vi "Digital input.vi"(8 "error in":errorcluster, 11 "DAQmx InPut Setting":T1) -> (0 "error out":errorcluster, 1 "Exit":bool)   [LabVIEW 2015]
uses:
  <vilib>/DAQmx/read.llb/DAQmx Read (Digital 1D Bool 1Chan 1Samp).vi
  <vilib>/DAQmx/create/channels.llb/DAQmx Create Channel (DI-Digital Input).vi
  Galobal variable_TI.vi
  <vilib>/DAQmx/miscellaneous.llb/DAQmx Fill In Error Info.vi
panel:
  in  "Count":i32
  out "Array":bool[](array[boolean])
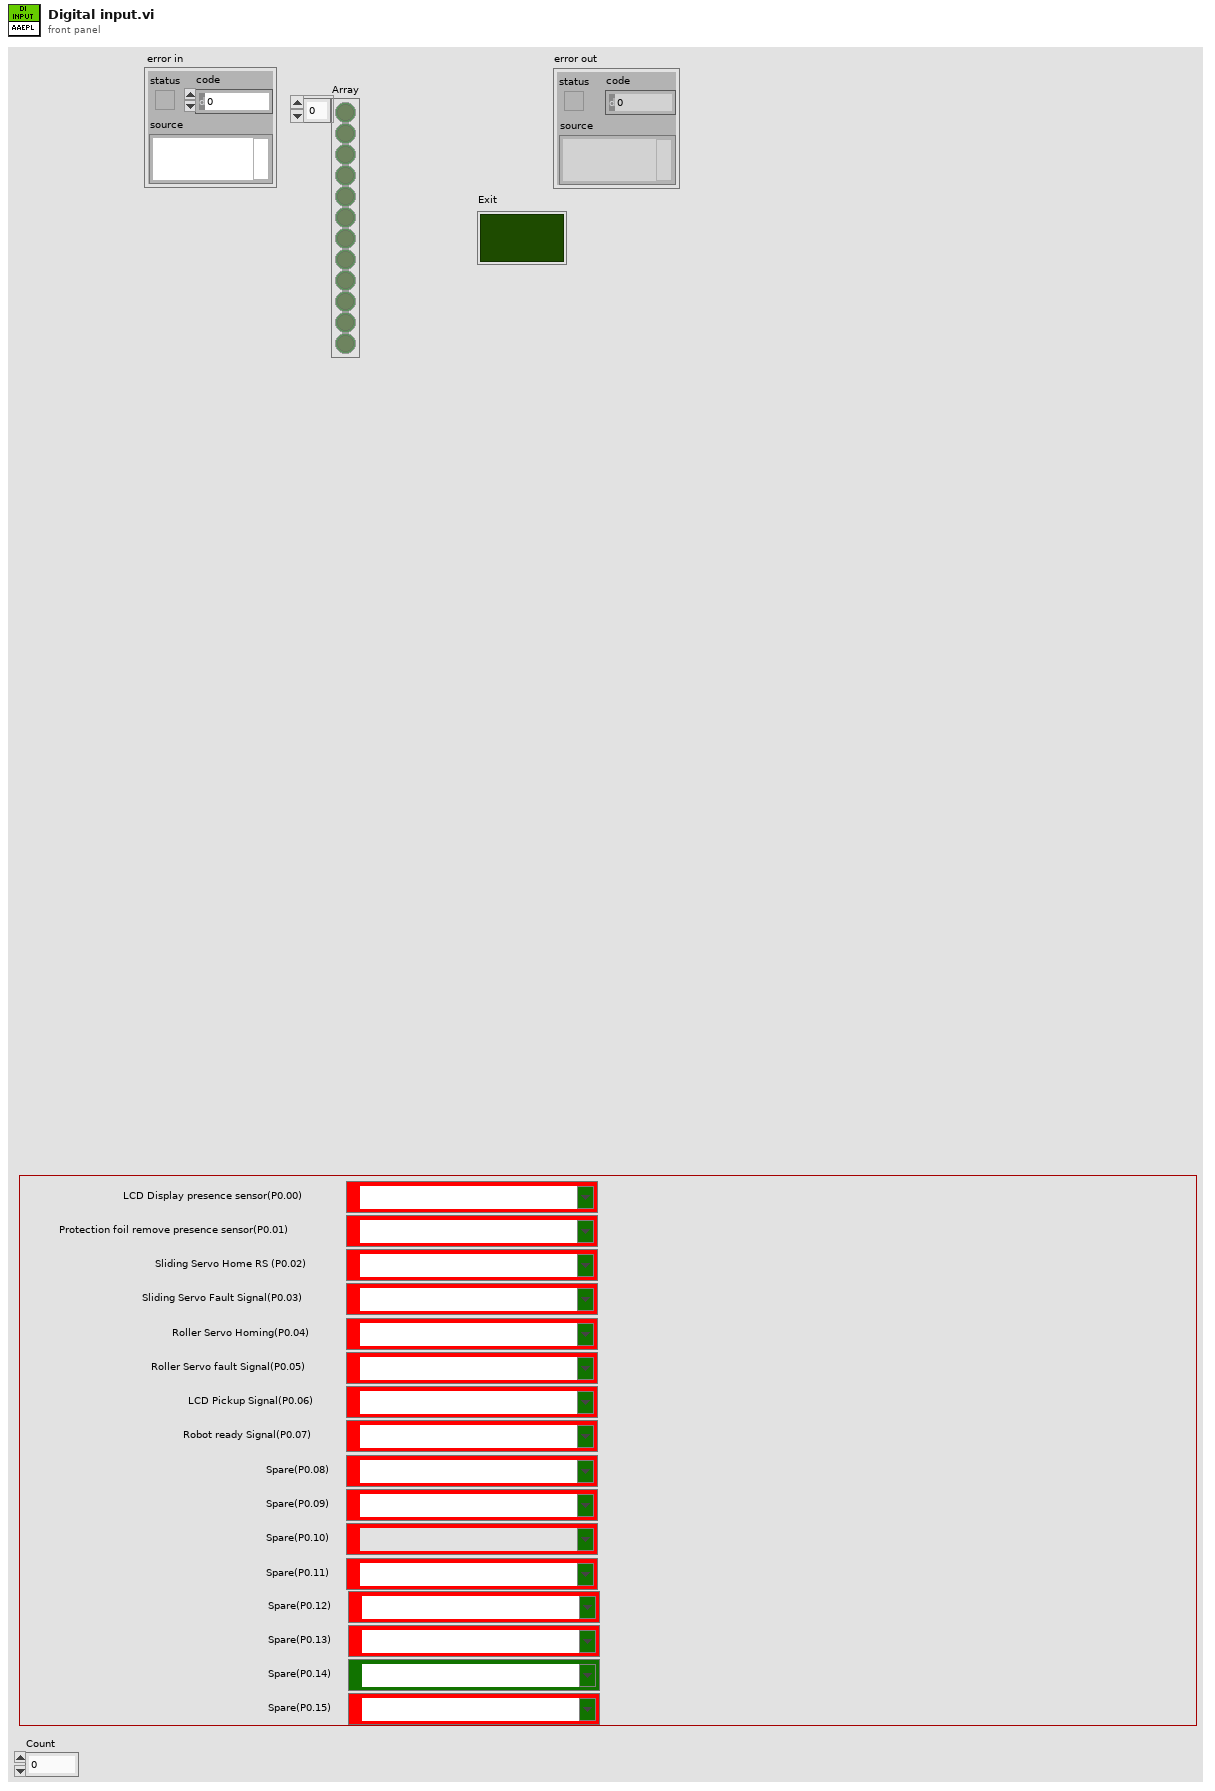
[diagram p1: front panel]
types:
  T1 = cluster{"DAQmx InPut_00":tag, "DAQmx InPut_01":tag, "DAQmx InPut_02":tag, "DAQmx InPut_03":tag, "DAQmx InPut_04":tag, "DAQmx InPut_05":tag, "DAQmx InPut_06":tag, "DAQmx InPut_07":tag, "DAQmx InPut_08":tag, "DAQmx InPut_09":tag, "DAQmx InPut_10":tag, "DAQmx InPut_11":tag, "DAQmx InPut_12":tag, "DAQmx InPut_13":tag, "DAQmx InPut_14":tag, "DAQmx InPut_15":tag}
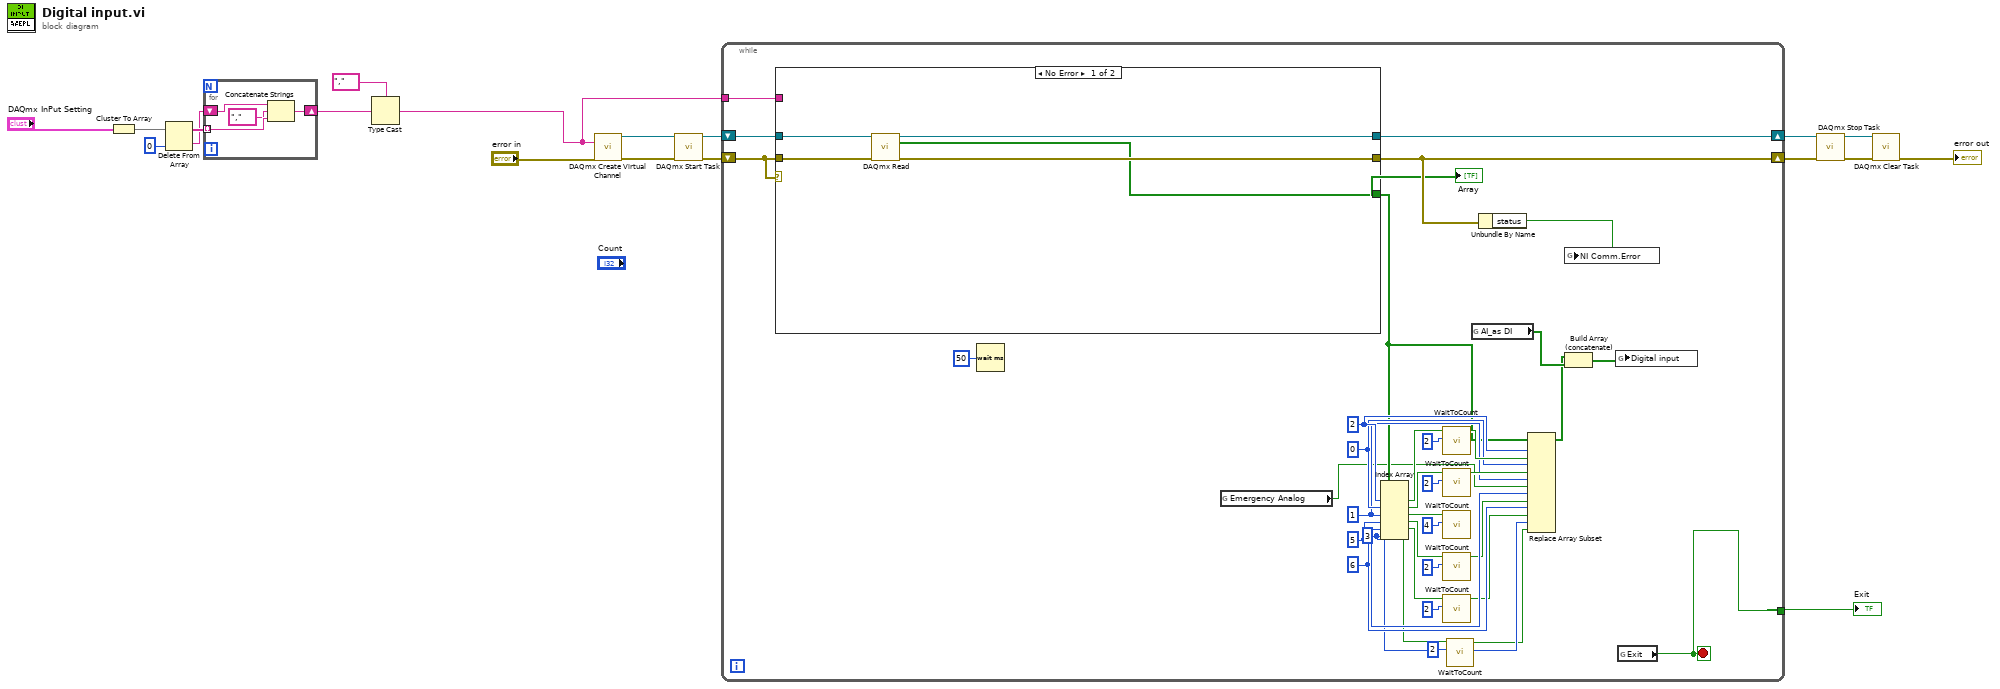
[diagram p0: block diagram]
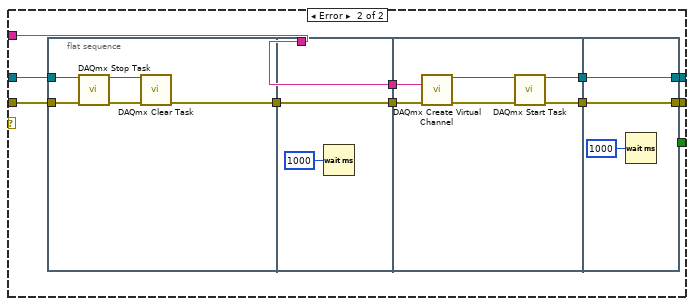
[diagram p2: hidden frame]
diagram:
  n1 = Cluster To Array(cluster="DAQmx InPut Setting") -> (array=w9:tag[])
  n2 = Delete From Array(array=w9, index=0) -> (deleted portion=w6:tag, array with subset deleted=w8:tag[])  [unwired: 1 in]
  n3 = for {
    tunnel: w8 -> [w22] mode=indexing
    shift-right: [w20] -> w4
    shift-left: w6 -> [w23]
    n4 = Concatenate Strings(w23, tag "," ("1."), w22) -> (w20:string)
  }
  n5 = Type Cast(type=tag "," ("1."), x=w4) -> (*(type *) &x=w3:tag)
  n6 = call-poly <vilib>:"DAQmx Create Virtual Channel.vi"("lines"=w3, "error in"="error in") -> ("task out"=w19:refnum<k21>, "error out"=w18:errorcluster)  [unwired: 3 in, 9 out]
  n7 = call <vilib>:"DAQmx Start Task.vi"("task/channels in"=w19, "error in"=w18) -> ("task out"=w16:refnum<k21>, "error out"=w17:errorcluster)  [unwired: 12 out]
  n8 = while {
    shift-right: [w51] -> w13
    shift-left: w17 -> [w59]
    shift-right: [w57] -> w12
    shift-left: w16 -> [w58]
    tunnel: w3 -> [w56]
    tunnel: [w55] -> w10
    stop <- w55 stop-if-true
    w28 = 3 ("index")
    w32 = 6 ("index")
    w38 = 5 ("index")
    w39 = 1 ("Count")
    w43 = 0 ("Count")
    w49 = 2 ("index")
    n9 = case shown="No Error" w59 {
      tunnel: w59 -> [w64 w73]
      tunnel: w58 -> [w63 w74]
      tunnel: [w62 w66] -> w51
      tunnel: [w61 w65] -> w57
      tunnel: w56 -> [_ w69]
      tunnel: [w60 _] -> w26
      frame No Error {
        n10 = call-poly <vilib>:"DAQmx Read.vi"("task/channels in"=w63, "error in"=w64) -> ("task out"=w61:refnum<k21>, "data"=w60:bool[], "error out"=w62:errorcluster)  [unwired: 1 in, 10 out]
      }
      frame Error {
        n11 = flat-sequence {
          tunnel: w74 -> [w77]
          tunnel: w73 -> [w76]
          tunnel: [w75] -> w72
          tunnel: w72 -> [w81]
          tunnel: [w81] -> w71
          tunnel: [w80] -> w70
          tunnel: w69 -> [w80]
          tunnel: w71 -> [w86]
          tunnel: w70 -> [w85]
          tunnel: [w84] -> w68
          tunnel: [w83] -> w67
          tunnel: w68 -> [w91]
          tunnel: w67 -> [w90]
          tunnel: [w91] -> w66
          tunnel: [w90] -> w65
          frame #0 {
            n12 = call <vilib>:"DAQmx Stop Task.vi"("task/channels in"=w77, "error in"=w76) -> ("task out"=w78:refnum<k21>, "error out"=w79:errorcluster)  [unwired: 12 in]
            n13 = call <vilib>:"DAQmx Clear Task.vi"("task in"=w78, "error in"=w79) -> ("error out"=w75:errorcluster)  [unwired: 13 in]
          }
          frame #1 {
            n14 = Wait (ms)(milliseconds to wait=u32 1000) -> ()  [unwired: 1 out]
          }
          frame #2 {
            n15 = call-poly <vilib>:"DAQmx Create Virtual Channel.vi"("lines"=w85, "error in"=w86) -> ("task out"=w87:refnum<k21>, "error out"=w88:errorcluster)  [unwired: 3 in, 9 out]
            n16 = call <vilib>:"DAQmx Start Task.vi"("task/channels in"=w87, "error in"=w88) -> ("task out"=w83:refnum<k21>, "error out"=w84:errorcluster)  [unwired: 12 out]
          }
          frame #3 {
            n17 = Wait (ms)(milliseconds to wait=u32 1000) -> ()  [unwired: 1 out]
          }
        }
      }
    }
    "Array" <- w26
    n18 = Wait (ms)(milliseconds to wait=u32 50) -> ()  [unwired: 1 out]
    n19 = global read "Galobal variable_TI.vi" "Emergency Analog"() -> (w25:bool)
    n20 = Index Array(array=w26, index #1=w49, index #2=w43, index #3=w39, index #4=w38, index #5=w32, index #6=w28) -> (element #1=w48:bool, element #2=w45:bool, element #3=w40:bool, element #4=w36:bool, element #5=w34:bool, element #6=w30:bool)
    n21 = call "WaitToCount.vi"("Count"=2, "Boolean-01"=w48) -> ("Boolean-01-Indicator"=w46:bool)  [unwired: 8 in, 1 out]
    n22 = call "WaitToCount.vi"("Count"=2, "Boolean-01"=w45) -> ("Boolean-01-Indicator"=w42:bool)  [unwired: 8 in, 1 out]
    n23 = call "WaitToCount.vi"("Count"=4, "Boolean-01"=w40) -> ()  [unwired: 8 in, 2 out]
    n24 = call "WaitToCount.vi"("Count"=2, "Boolean-01"=w36) -> ("Boolean-01-Indicator"=w37:bool)  [unwired: 8 in, 1 out]
    n25 = call "WaitToCount.vi"("Count"=2, "Boolean-01"=w34) -> ("Boolean-01-Indicator"=w31:bool)  [unwired: 8 in, 1 out]
    n26 = call "WaitToCount.vi"("Count"=2, "Boolean-01"=w30) -> ("Boolean-01-Indicator"=w27:bool)  [unwired: 8 in, 1 out]
    n27 = global read "Galobal variable_TI.vi" "AI_as DI"() -> (w53:bool[])
    n28 = Unbundle By Name(w51) -> ("status"=w50:bool)
    n29 = Replace Array Subset(array=w26, new element #1=w46, index #1=w49, new element #2=w42, index #2=w43, new element #3=w25, index #3=w39, new element #4=w37, index #4=w38, new element #5=w31, index #5=w32, new element #6=w27, index #6=w28) -> (w24:bool[])
    n30 = global write "Galobal variable_TI.vi" "NI Comm.Error"(w50) -> ()
    n31 = Build Array (concatenate)(w24, w53) -> (w54:bool[])
    n32 = global write "Galobal variable_TI.vi" "Digital input"(w54) -> ()
    n33 = global read "Galobal variable_TI.vi" "Exit"() -> (w55:bool)
  }
  "Exit" <- w10
  n34 = call <vilib>:"DAQmx Stop Task.vi"("task/channels in"=w12, "error in"=w13) -> ("task out"=w14:refnum<k21>, "error out"=w15:errorcluster)  [unwired: 12 in]
  n35 = call <vilib>:"DAQmx Clear Task.vi"("task in"=w14, "error in"=w15) -> ("error out"=→"error out":errorcluster)  [unwired: 13 in]
